vi "PostInstall.vi"(10 "Variant":variant) -> (0 "error out":errorcluster)   [LabVIEW 2017]
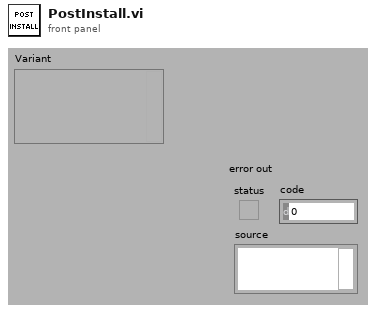
[diagram p1: front panel]
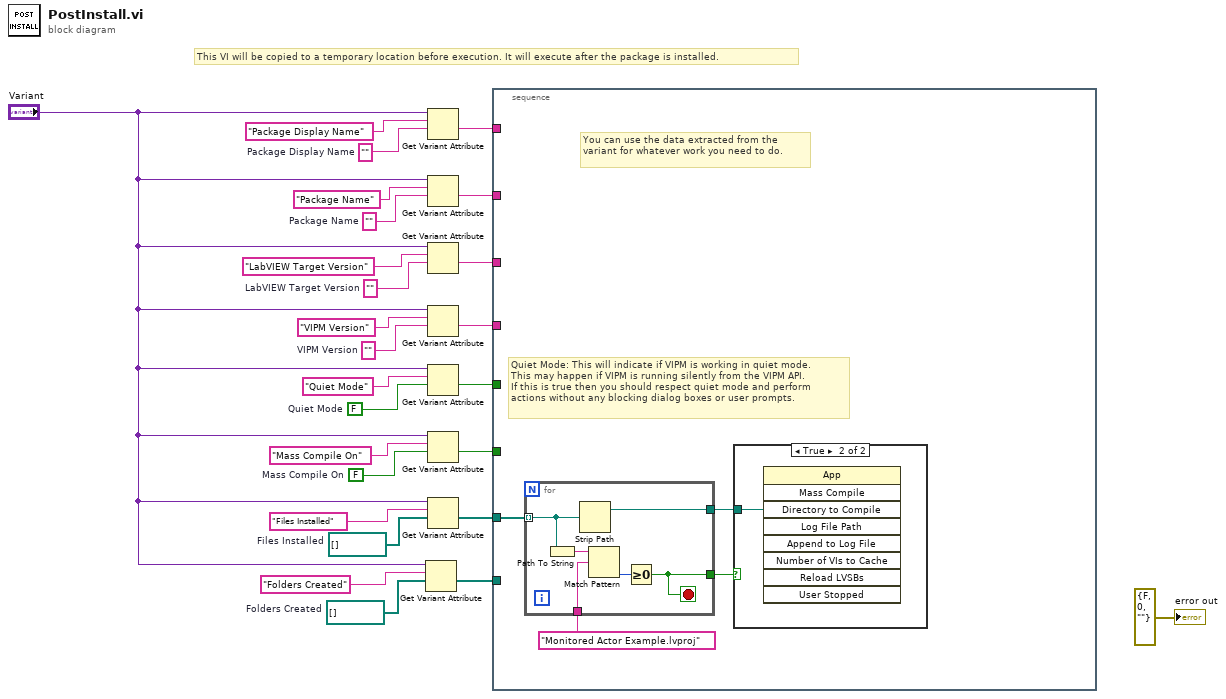
[diagram p0: block diagram]
diagram:
  w1 = path[] []  # Folders Created
  w2 = path[] []  # Files Installed
  w8 = FALSE  # Mass Compile On
  w9 = ""  # Package Display Name
  w16 = FALSE  # Quiet Mode
  w19 = ""  # VIPM Version
  w21 = ""  # LabVIEW Target Version
  w23 = ""  # Package Name
  # "This VI will be copied to a temporary location before execution. It will execute after the package is installed."
  n1 = Get Variant Attribute(Variant="Variant", name="Folders Created", default value (empty Variant)=w1) -> (value=w6:path[])  [unwired: 1 in, 3 out]
  n2 = Get Variant Attribute(Variant="Variant", name="Package Display Name", default value (empty Variant)=w9) -> (value=w15:string)  [unwired: 1 in, 3 out]
  n3 = Get Variant Attribute(Variant="Variant", name="Package Name", default value (empty Variant)=w23) -> (value=w14:string)  [unwired: 1 in, 3 out]
  n4 = Get Variant Attribute(Variant="Variant", name="LabVIEW Target Version", default value (empty Variant)=w21) -> (value=w13:string)  [unwired: 1 in, 3 out]
  n5 = Get Variant Attribute(Variant="Variant", name="VIPM Version", default value (empty Variant)=w19) -> (value=w12:string)  [unwired: 1 in, 3 out]
  n6 = Get Variant Attribute(Variant="Variant", name="Quiet Mode", default value (empty Variant)=w16) -> (value=w11:bool)  [unwired: 1 in, 3 out]
  n7 = Get Variant Attribute(Variant="Variant", name="Mass Compile On", default value (empty Variant)=w8) -> (value=w10:bool)  [unwired: 1 in, 3 out]
  n8 = Get Variant Attribute(Variant="Variant", name="Files Installed", default value (empty Variant)=w2) -> (value=w5:path[])  [unwired: 1 in, 3 out]
  n9 = stacked-sequence {
    tunnel: w15 -> [_]
    tunnel: w14 -> [_]
    tunnel: w13 -> [_]
    tunnel: w12 -> [_]
    tunnel: w11 -> [_]
    tunnel: w10 -> [_]
    tunnel: w5 -> [w30]
    tunnel: w6 -> [_]
    frame #0 {
      # "Quiet Mode: This will indicate if VIPM is working in quiet mode.\nThis may happen if VIPM is running silently from the VIPM API.\nIf this is true then you should respect quiet mode and perform\nactions without any blocking dialog boxes or user prompts."
      # "You can use the data extracted from the variant for whatever work you need to do."
      n10 = for {
        tunnel: w30 -> [w34] mode=indexing
        tunnel: "Monitored Actor Example.lvproj" ("regular expression") -> [w36]
        tunnel: [w33] -> w28
        tunnel: [w32] -> w27
        stop <- w33 stop-if-true
        n11 = Path To String(path=w34) -> (string=w37:string)
        n12 = Strip Path(path=w34) -> (stripped path=w32:path)  [unwired: 1 out]
        n13 = Match Pattern(string=w37, regular expression=w36) -> (offset past match=w35:i32)  [unwired: 1 in, 3 out]
        n14 = Greater Or Equal To 0?(x=w35) -> (x >= 0?=w33:bool)
      }
      n15 = case shown="True" w28 {
        tunnel: w27 -> [_ w31]
        frame False {
        }
        frame True {
          n16 = invoke class="App" method="Mass Compile"("Directory to Compile"=w31) -> ()  [unwired: 8 in, 9 out]
        }
      }
    }
  }
  "error out" <- errorcluster {"status"=FALSE, "code"=0, "source"=""} ("error out")
